vi "WaitForEdge.vi"() -> ()   [LabVIEW 2014]
doc: "This example VI demonstrates the use of GPIO interrupts to wait for an edge event on multiple inputs. \n\nTo use this VI simply wire an appropriate LED between a GPIO channel and Ground. Supply the pin number (default = GPIO 24) to the Output channel control. Likewise wire a simple button to multiple different GPIO channels and supply the pin numbers to the Input channels control.\n\nBroadcom numbering for the GPIO pins is assumed by this VI.\n\nAfter wiring the circuit, deploy the VI to the Raspberry Pi and run it. When you push and/or release one of the buttons depending on the Edge setting, an event will be triggered and the output channel will be toggled. Multiple toggles with a single press are most likely the result of switch bouncing."
uses:
  controls/IO_Direction.ctl
panel:
  out "error out":errorcluster
  out "Value":bool
  in  "Stop":bool
  in  "Edge":enum16{"Rising", "Falling", "Both"}(ring)
  in  "Output channel":i32=24
  in  "Input channels":i32[](array[numeric])=[25, 26]
  # "Wire Buttons to GPIO Input Channels\nWire LED to Output Channel\n\nEdge detection toggles LED"
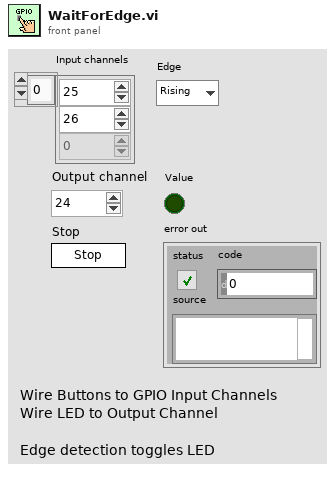
[diagram p1: front panel]
types:
  T1 = typedef "IO_Direction.ctl" = enum16{"Input", "Output"}
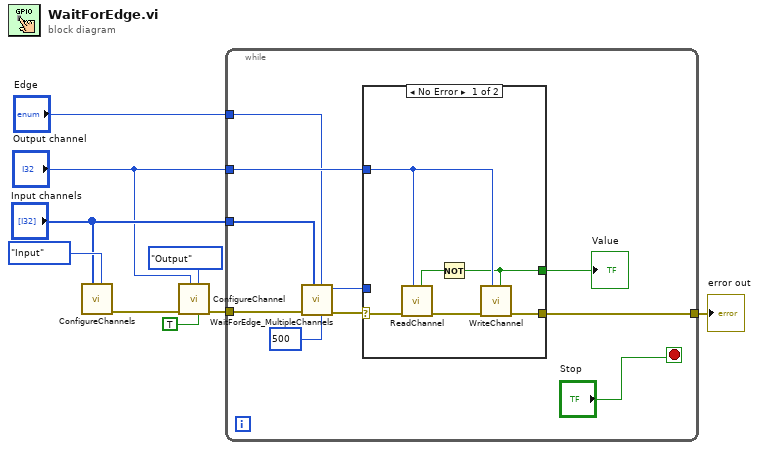
[diagram p0: block diagram]
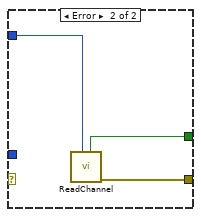
[diagram p2: hidden frame]
diagram:
  n1 = call "ConfigureChannels.vi"("Direction"=IO_Direction."Input", "Channels"="Input channels") -> ("error out"=w5:errorcluster)  [unwired: 9 in]
  n2 = call "ConfigureChannel.vi"("Initial value"=TRUE, "Direction"=IO_Direction."Output", "Channel"="Output channel", "error in"=w5) -> ("error out"=w4:errorcluster)  [unwired: 7 in]
  n3 = while {
    tunnel: w4 -> [w19]
    tunnel: "Input channels" -> [w15]
    tunnel: "Output channel" -> [w14]
    tunnel: "Edge" -> [w13]
    tunnel: [w11] -> w1
    stop <- "Stop" stop-if-true
    n4 = call "WaitForEdge_MultipleChannels.vi"("Timeout (msec)"=500, "Edge"=w13, "Channels"=w15, "error in"=w19) -> ("error out"=w17:errorcluster, "Channel out"=w16:i32)  [unwired: 6 in]
    n5 = case shown="No Error" w17 {
      selector: w17 -> [w25 _]
      tunnel: w16 -> [_ _]
      tunnel: w14 -> [w21 w26]
      tunnel: [w23 w28] -> w11
      tunnel: [w20 w27] -> w12
      frame No Error {
        n6 = call "ReadChannel.vi"("Channel"=w21, "error in"=w25) -> ("error out"=w24:errorcluster, "Value"=w22:bool)  [unwired: 6 in]
        n7 = Not(x=w22) -> (.not. x?=w20:bool)
        n8 = call "WriteChannel.vi"("Value"=w20, "Channel"=w21, "error in"=w24) -> ("error out"=w23:errorcluster)  [unwired: 6 in]
      }
      frame Error {
        n9 = call "ReadChannel.vi"("Channel"=w26) -> ("error out"=w28:errorcluster, "Value"=w27:bool)  [unwired: 7 in]
      }
    }
    "Value" <- w12
  }
  "error out" <- w1
